vi "Save attributes.vi"(7 "Save data?":bool, 8 "error in (no error)":errorcluster, 9 "Timestep":dbl, 10 "coefficient info":T1(array[cluster]), 11 "Refnum in":T2) -> (0 "error out":errorcluster, 3 "Refnum out":T2)   [LabVIEW 2018]
uses:
  <vilib>/UPVI/lvhdf5/library.llb/HDF5 Ref.ctl
  <vilib>/UPVI/lvhdf5/attribute.llb/LVH5A Operation.ctl
  <vilib>/Utility/VariantDataType/GetClusterInfo.vi
  <vilib>/Utility/VariantDataType/GetTypeInfo.vi
  <vilib>/UPVI/lvhdf5/attribute.llb/Write Multiple Attributes.vi
  <vilib>/UPVI/lvhdf5/attribute.llb/LVH5 Write Attributes.xnode
  <vilib>/UPVI/lvhdf5/attribute.llb/Cluster to Attribute Array.xnode
  <vilib>/Utility/VariantDataType/VariantType.lvlib
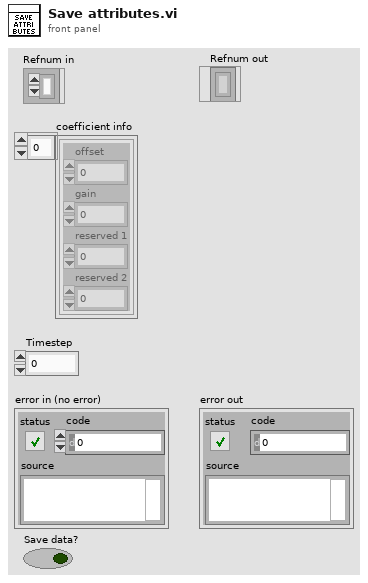
[diagram p1: front panel]
types:
  T1 = cluster{"offset":dbl, "gain":dbl, "reserved 1":dbl, "reserved 2":dbl}[]
  T2 = typedef "HDF5 Ref.ctl" = refnum<k1>
  T3 = cluster{"offset":dbl, "timestep":dbl, "gain":dbl}
  T4 = typedef "LVH5A Operation.ctl" = enum16{"open", "replace", "create", "open or create", "create or replace", "create or replace with confirmation"}
  T5 = cluster{"offset":dbl, "gain":dbl, "reserved 1":dbl, "reserved 2":dbl}
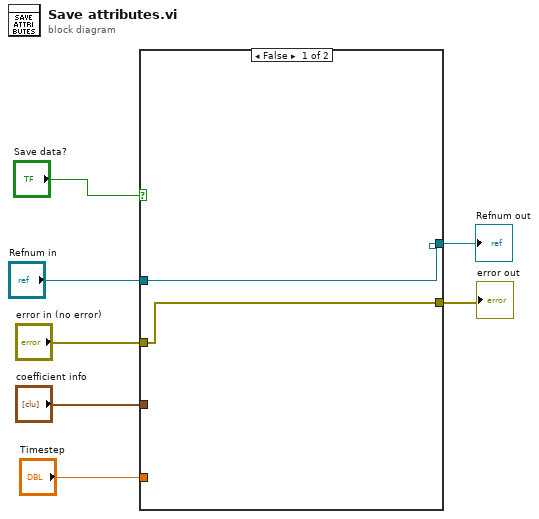
[diagram p0: block diagram]
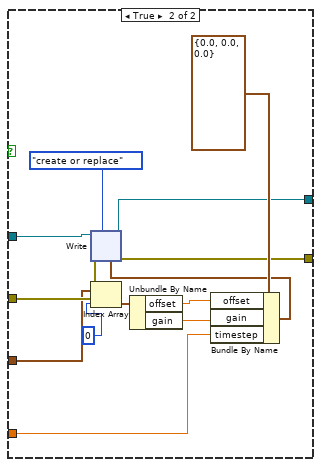
[diagram p2: hidden frame]
diagram:
  n1 = case shown="False" "Save data?" {
    tunnel: "Timestep" -> [_ w22]
    tunnel: [w9 w16] -> w6
    tunnel: [w8 w15] -> w5
    tunnel: "error in (no error)" -> [w8 w14]
    tunnel: "Refnum in" -> [w9 w13]
    tunnel: "coefficient info" -> [_ w12]
    frame False {
    }
    frame True {
      n2 = Index Array(array=w12, index=0) -> (element=w17:T5)
      n3 = Unbundle By Name(w17) -> ("offset"=w18:dbl, "gain"=w19:dbl)
      n4 = Bundle By Name(cluster=T3 {"offset"=0.0, "timestep"=0.0, "gain"=0.0} ("input cluster"), "offset"=w18, "gain"=w19, "timestep"=w22) -> (w20:T3)
      n5 = xnode "Write"("HDF5 Ref"=w13, "error in (no error)"=w14, "operation (create or replace)"=LVH5A_Operation."create or replace", "Value(s)"=w20) -> ("HDF5 Ref out"=w16:T2, "error out"=w15:errorcluster)  [unwired: 1 in]
    }
  }
  "Refnum out" <- w6
  "error out" <- w5
